vi "Mixer.GetWindowState.vi"() -> (0 "state":string)   [LabVIEW 2020]
panel:
  out "error out":errorcluster
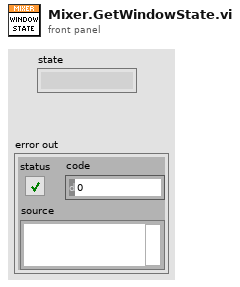
[diagram p1: front panel]
types:
  T1 = enum32{"Invalid", "Standard", "Closed", "Hidden", "Minimized", "Maximized"}
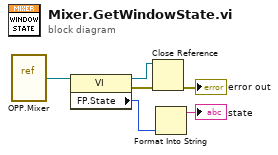
[diagram p0: block diagram]
diagram:
  n1 = vi-ref "OPP.Mixer.vi"() -> (w6:refnum<vi>)
  n2 = property class="VI"(reference=w6) -> (reference out=w3:refnum<vi>, error out=w4:errorcluster, "FP.State"=w2:T1)  [unwired: 1 in]
  n3 = Close Reference(reference=w3, error in (no error)=w4) -> (error out=→"error out":errorcluster)
  n4 = Format Into String(w2) -> (resulting string=→"state":string)  [unwired: 3 in, 1 out]
